vi "P4CMD Undo Check Out.vi"(7 "advanced options":variant, 8 "error in (no error)":errorcluster, 10 "files":path[](array[path]), 11 "source control reference in":T1) -> (0 "error out":errorcluster, 1 "dialog box cancelled?":bool, 2 "status message":string, 3 "source control reference out":T1)   [LabVIEW 2017, in "NI_SCC_P4CMD.lvlib"]
uses:
  <vilib>/SourceControl/Providers/P4CMD/NI_SCC_P4CMD.lvlib
  <vilib>/SourceControl/sccapi/SCCAPI Refnum.ctl
  <vilib>/SourceControl/Providers/P4CMD/P4CMD Operations.ctl
  <vilib>/SourceControl/support/SCCSup Message Strings GLBL.vi
  <vilib>/SourceControl/sccapi/NI_SCC.lvlib
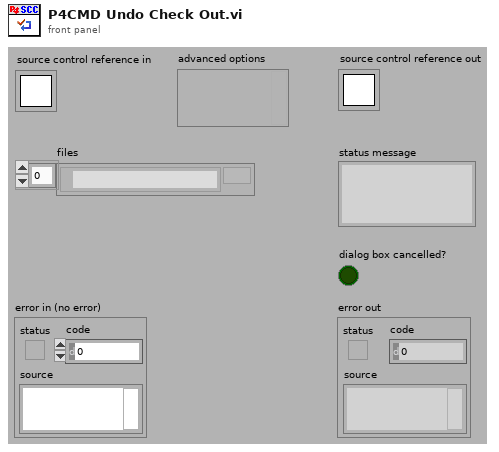
[diagram p1: front panel]
types:
  T1 = typedef "NI_SCC.lvlib/SCCAPI Refnum.ctl" = refnum<k1>
  T2 = typedef "NI_SCC_P4CMD.lvlib/P4CMD Operations.ctl" = enum16{"get all clients", "get all users", "describe changelist", "sync from depot", "open for edit", "submit to depot", "revert", "add to depot", "remove from depot", "print files revisions", "compare client file", "print depot file contents", "list opened files", "get file info", "lock files", "edit changelist spec", "info", "set variables"}
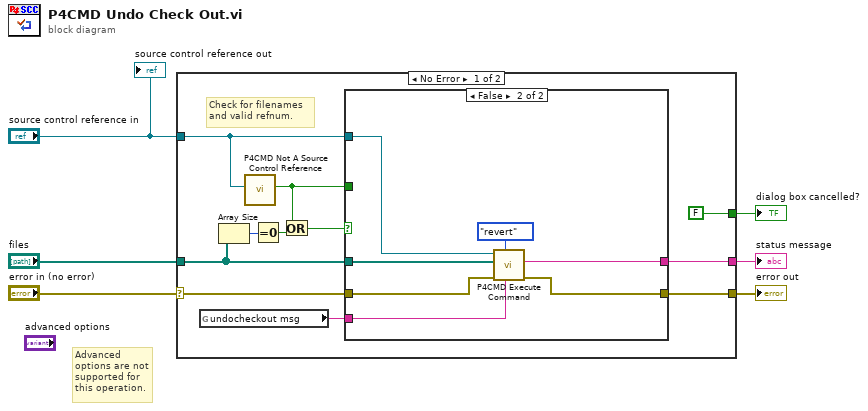
[diagram p0: block diagram]
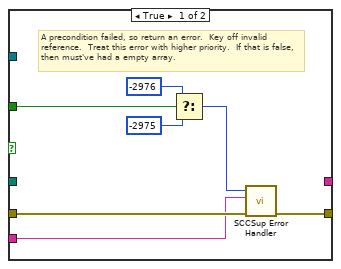
[diagram p2: hidden frame]
diagram:
  # "Advanced options are not supported for this operation."
  n1 = case shown="No Error" "error in (no error)" {
    selector: "error in (no error)" -> [w10 w32]
    tunnel: [w8 w32] -> w5
    tunnel: "source control reference in" -> [w15 _]
    tunnel: [w9 _] -> w3
    tunnel: "files" -> [w14 _]
    tunnel: [FALSE _] -> w1
    frame No Error {
      # "Check for filenames and valid refnum."
      n2 = global read "SCCSup Message Strings GLBL.vi" "undocheckout msg"() -> (w7:string)
      n3 = Array Size(array=w14) -> (size(s)=w16:i32)
      n4 = call <vilib>:"P4CMD Not A Source Control Reference.vi"("source control reference in"=w15) -> ("not a source control reference?"=w12:bool)  [unwired: 9 in, 1 out]
      n5 = Equal To 0?(x=w16) -> (x = 0?=w17:bool)
      n6 = Or(x=w12, y=w17) -> (x .or. y?=w13:bool)
      n7 = case shown="False" w13 {
        tunnel: w15 -> [_ w28]
        tunnel: w14 -> [_ w27]
        tunnel: w12 -> [w22 _]
        tunnel: w10 -> [w20 w29]
        tunnel: [_ w30] -> w9
        tunnel: [w19 w26] -> w8
        tunnel: w7 -> [w18 w25]
        frame True {
          # "A precondition failed, so return an error.  Key off invalid reference.  Treat this error with higher priority.  If that is false, then must've had a empty array."
          n8 = Select(t=-2976 ("result"), s=w22, f=-2975 ("result")) -> (s? t:f=w21:i32)
          n9 = call <vilib>:"SCCSup Error Handler.vi"("error in (no error)"=w20, "operation message"=w18, "scc error code"=w21) -> ("error out"=w19:errorcluster)  [unwired: 8 in]
        }
        frame False {
          n10 = call <vilib>:"P4CMD Execute Command.vi"("operation message"=w25, "p4 operation"=P4CMD_Operations."revert", "error in (no error)"=w29, "files"=w27, "source control reference in"=w28) -> ("error out"=w26:errorcluster, "command information"=w30:string)  [unwired: 4 in, 1 out]
        }
      }
    }
    frame Error {
    }
  }
  "error out" <- w5
  "status message" <- w3
  "dialog box cancelled?" <- w1
  "source control reference out" <- "source control reference in"
